vi "Raw to I32 Encoder.vi"(6 "step threshold":i32=10000 format="%x", 8 "enable step filter (True)":bool=TRUE, 9 "Low Byte":u8, 10 "Mid Byte":u8, 11 "High Byte":u8) -> (3 "out":i32)   [LabVIEW 2016]
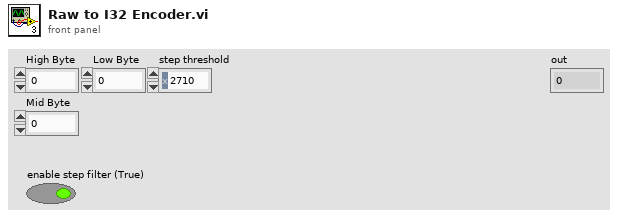
[diagram p1: front panel]
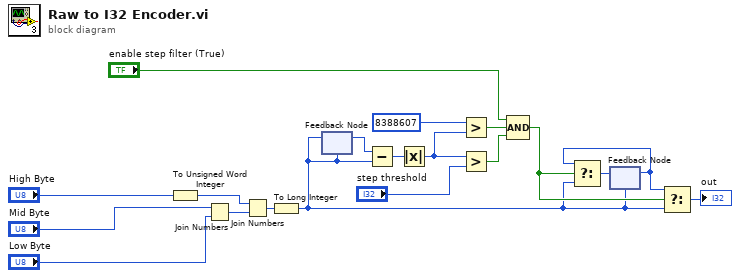
[diagram p0: block diagram]
diagram:
  n1 = To Unsigned Word Integer(number="High Byte") -> (unsigned 16bit integer=w13:u16)
  n2 = Join Numbers(hi="Mid Byte", lo="Low Byte") -> ((hi.lo)=w18:u16)
  n3 = Join Numbers(hi=w13, lo=w18) -> ((hi.lo)=w19:u32)
  n4 = To Long Integer(number=w19) -> (32bit integer=w6:i32)
  n5 = feedback #1(w6) -> (w7:i32)
  n6 = feedback-in #1(w6) -> ()
  n7 = Subtract(x=w7, y=w6) -> (x-y=w9:i32)
  n8 = Absolute Value(x=w9) -> (abs(x)=w3:i32)
  n9 = Greater?(x=8388607, y=w3) -> (0:w1:bool)
  n10 = Greater?(x=w3, y="step threshold") -> (0:w5:bool)
  n11 = Compound Arithmetic op=AND("enable step filter (True)", w1, w5) -> (w10:bool)
  n12 = feedback #2(w6) -> (w11:i32)
  n13 = Select(t=w11, s=w10, f=w6) -> (s? t:f=w12:i32)
  n14 = feedback-in #2(w12) -> ()
  n15 = Select(t=w11, s=w10, f=w6) -> (s? t:f=→"out":i32)
